vi "纳清_第三点原始光强值写入.vi"(7 "探头":T1(ring), 8 "error in (no error)":errorcluster caption="错误输入（无错误）", 10 "数值":u16, 11 "MB session in":refnum<class "MB_Master.lvclass">) -> (0 "error out":errorcluster caption="错误输出", 3 "MB session out":refnum<class "MB_Master.lvclass">)   [LabVIEW 2016, in "斯坦道多参数.lvlib"]
uses:
  <vilib>/Plasmionique/MB Master/MB Master.lvlib
  <vilib>/Plasmionique/MB Master/MB_Master/MB_Master.lvclass
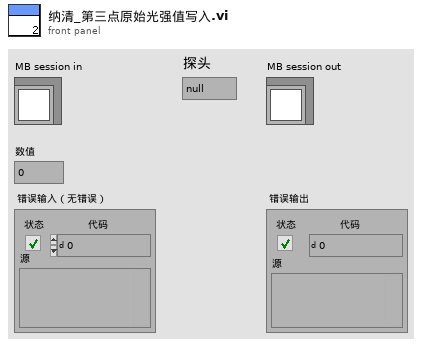
[diagram p1: front panel]
types:
  T1 = enum16{"null", "pH", "DO", "浊度", "电导率", "叶绿素a", "藻密度", "氨氮"}
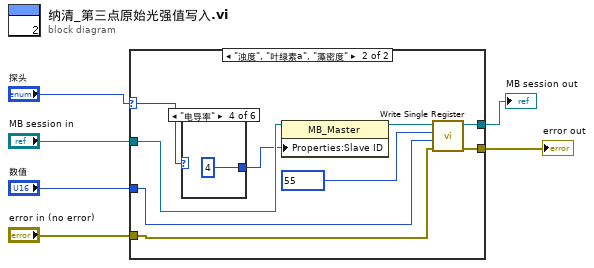
[diagram p0: block diagram]
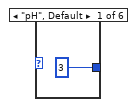
[diagram p3: hidden frame]
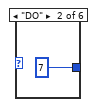
[diagram p4: hidden frame]
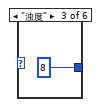
[diagram p5: hidden frame]
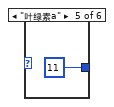
[diagram p6: hidden frame]
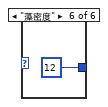
[diagram p7: hidden frame]
diagram:
  n1 = case shown="\"浊度\", \"叶绿素a\", \"藻密度\"" "探头" {
    selector: "探头" -> [_ w9]
    tunnel: "error in (no error)" -> [w7 w16]
    tunnel: [w7 w15] -> w5
    tunnel: "MB session in" -> [w8 w13]
    tunnel: [w8 w12] -> w3
    tunnel: "数值" -> [_ w10]
    frame "pH", Default {
    }
    frame "浊度", "叶绿素a", "藻密度" {
      n2 = case shown="\"电导率\"" w9 {
        tunnel: [3 7 8 4 11 12] -> w11
        frame "pH", Default {
        }
        frame "DO" {
        }
        frame "浊度" {
        }
        frame "电导率" {
        }
        frame "叶绿素a" {
        }
        frame "藻密度" {
        }
      }
      n3 = property class="MB_Master"(reference=w13, "Properties:Slave ID"=w11) -> (reference out=w14:refnum<class "MB_Master.lvclass">)  [unwired: 1 in, 1 out]
      n4 = call <vilib>:"Write Single Register.vi"("error in (no error)"=w16, "value"=w10, "address"=u16 55 ("starting address"), "MB session in"=w14) -> ("error out"=w15:errorcluster, "MB session out"=w12:refnum<class "MB_Master.lvclass">)  [unwired: 6 in]
    }
  }
  "error out" <- w5
  "MB session out" <- w3
